vi "StripOldFIlePath.vi"(4 "Path2Split":path=path "C:/Users/h2odial/WVD-MCSupdate/WVDNewArchitectureUpdate/WVD_Architecture_Update/Data/MCS/20190222/MCSPower_20190222_214124.txt") -> (0 "EndString":string, 1 "FileName":string="MCSPower_20190222_214124.txt", 2 "FullPath":string="C:\\Users\\h2odial\\WVD-MCSupdate\\WVDNewArchitectureUpdate\\WVD_Architecture_Update\\Data\\MCS\\20190222\\")   [LabVIEW 2012]
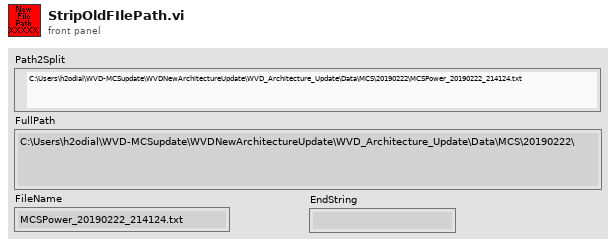
[diagram p1: front panel]
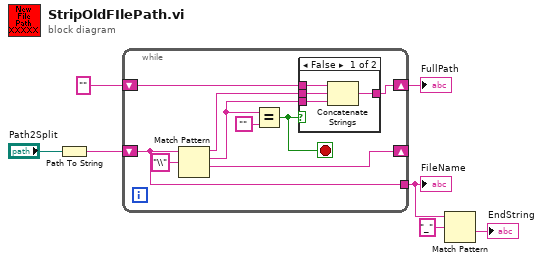
[diagram p0: block diagram]
diagram:
  n1 = Path To String(path="Path2Split") -> (string=w6:string)
  n2 = while {
    shift-right: [w13] -> _
    shift-left: w6 -> [w10]
    shift-right: [w9] -> w4
    shift-left: "" -> [w14]
    tunnel: [w10] -> w3
    stop <- w8 stop-if-true
    n3 = Match Pattern(string=w10, regular expression="\\") -> (before substring=w15:string, match substring=w12:string, after substring=w13:string)  [unwired: 1 in, 1 out]
    n4 = Equal?(x=w12, y="") -> (x = y?=w8:bool)
    n5 = case shown="False" w8 {
      tunnel: w15 -> [w20 _]
      tunnel: [w19 w21] -> w9
      tunnel: w14 -> [w18 w21]
      tunnel: w12 -> [w17 _]
      frame False {
        n6 = Concatenate Strings(w18, w20, w17) -> (w19:string)
      }
      frame True {
      }
    }
  }
  "FullPath" <- w4
  "FileName" <- w3
  n7 = Match Pattern(string=w3, regular expression="_") -> (after substring=→"EndString":string)  [unwired: 1 in, 3 out]
